vi "Get Reference.vi"(8 "Error In":errorcluster, 9 "Subpanel Ref":refnum<vi>, 11 "Sample Test Template in":refnum<class "Sample Test Template.lvclass">) -> (0 "Error Out":errorcluster, 3 "Sample Test Template out":refnum<class "Sample Test Template.lvclass">)   [LabVIEW 2020, in "Sample Test Template.lvclass"]
uses:
  Sample Test Template.lvclass
  D:/SDLC/Class/Test/Parent/Test.lvclass
  Parent/Typedef/LV2 Control.ctl
  Device/Parent/Device.lvclass
  Parent/Test.lvclass
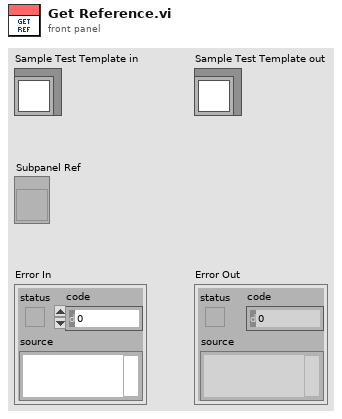
[diagram p1: front panel]
types:
  T1 = typedef "Test.lvclass/LV2 Control.ctl" = enum16{"Home", "Mode", "Config", "Status", "Read"}
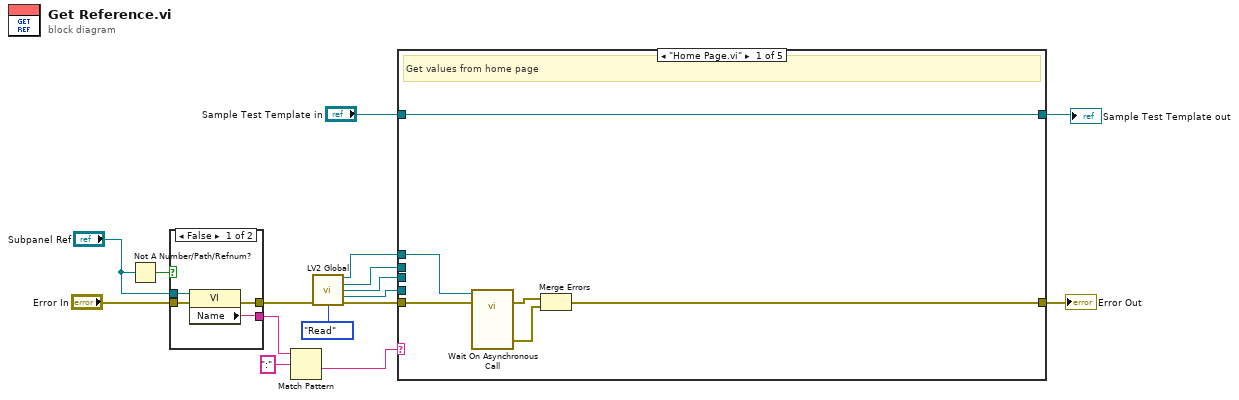
[diagram p0: block diagram]
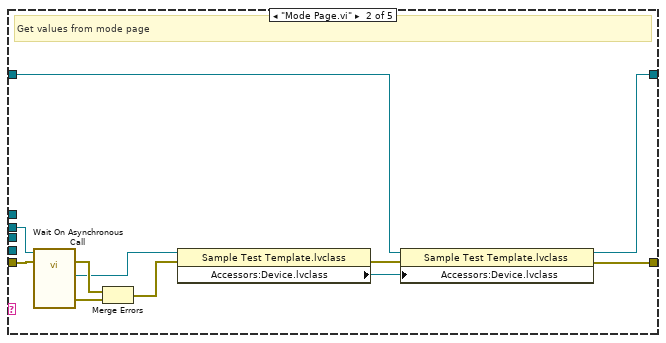
[diagram p2: hidden frame]
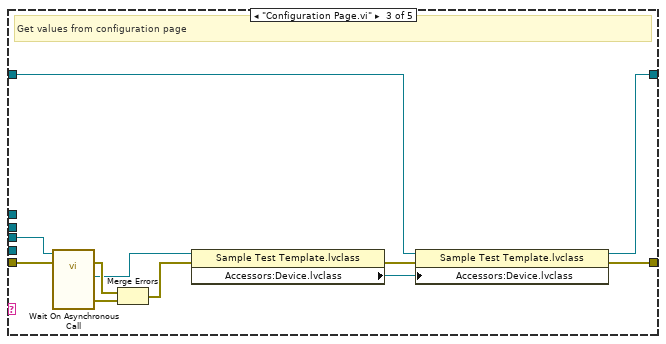
[diagram p3: hidden frame]
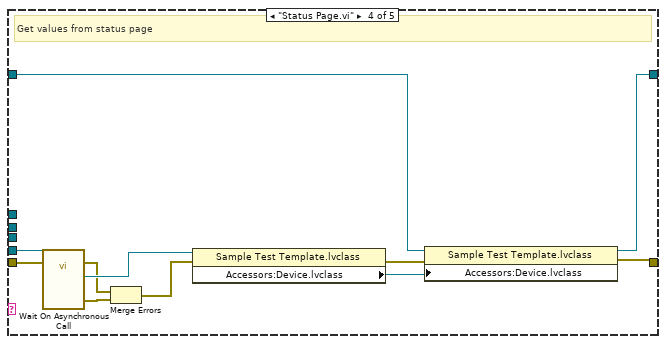
[diagram p4: hidden frame]
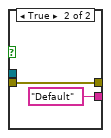
[diagram p6: hidden frame]
diagram:
  n1 = Not A Number/Path/Refnum?(number/path/refnum="Subpanel Ref") -> (NaN/Path/Refnum?=w16:bool)
  n2 = case shown="False" w16 {
    tunnel: "Error In" -> [w20 w22]
    tunnel: [w19 w22] -> w7
    tunnel: [w18 "Default" ("Name")] -> w15
    tunnel: "Subpanel Ref" -> [w17 _]
    frame False {
      n3 = property class="VI"(reference=w17, error in=w20) -> (error out=w19:errorcluster, "Name"=w18:string)  [unwired: 1 out]
    }
    frame True {
    }
  }
  n4 = Match Pattern(string=w15, regular expression=":") -> (after substring=w13:string)  [unwired: 1 in, 3 out]
  n5 = call "LV2 Global.vi"("Error In"=w7, "Enum"=LV2_Control."Read") -> ("Home Ref"=w1:refnum<vi>, "Mode Ref"=w4:refnum<vi>, "Configuration Ref"=w3:refnum<vi>, "Status Ref"=w2:refnum<vi>, "Error Out"=w6:errorcluster)  [unwired: 9 in]
  n6 = case shown="\"Home Page.vi\"" w13 {
    tunnel: w6 -> [w26 w39 w47 w61 w63]
    tunnel: [w23 w35 w43 w54 w63] -> w10
    tunnel: [w28 w30 w41 w52 w62] -> w8
    tunnel: "Sample Test Template in" -> [w28 w31 w42 w53 w62]
    tunnel: w4 -> [_ w29 _ _ _]
    tunnel: w3 -> [_ _ w40 _ _]
    tunnel: w2 -> [_ _ _ w51 _]
    tunnel: w1 -> [w27 _ _ _ _]
    frame "Home Page.vi" {
      # "Get values from home page"
      n7 = call-by-ref "Wait On Asynchronous Call"(reference=w27, error in=w26) -> (error out=w25:errorcluster, "Error Out"=w24:errorcluster)  [unwired: 14 in, 2 out]
      n8 = Merge Errors(w25, w24) -> (w23:errorcluster)
    }
    frame "Mode Page.vi" {
      # "Get values from mode page"
      n9 = call-by-ref "Wait On Asynchronous Call"(reference=w29, error in=w39) -> (error out=w38:errorcluster, 0:"error out"=w37:errorcluster, "Sample Test Template out"=w33:refnum<class "Sample Test Template.lvclass">)  [unwired: 10 in, 1 out]
      n10 = Merge Errors(w38, w37) -> (w36:errorcluster)
      n11 = property class="Sample Test Template.lvclass"(reference=w33, error in=w36) -> (error out=w34:errorcluster, "Accessors:Device.lvclass"=w32:refnum<class "Device.lvclass">)  [unwired: 1 out]
      n12 = property class="Sample Test Template.lvclass"(reference=w31, error in=w34, "Accessors:Device.lvclass"=w32) -> (reference out=w30:refnum<class "Sample Test Template.lvclass">, error out=w35:errorcluster)
    }
    frame "Configuration Page.vi" {
      # "Get values from configuration page"
      n13 = call-by-ref "Wait On Asynchronous Call"(reference=w40, error in=w47) -> (error out=w46:errorcluster, "Error Out"=w45:errorcluster, "Sample Test Template out"=w44:refnum<class "Sample Test Template.lvclass">)  [unwired: 10 in, 1 out]
      n14 = Merge Errors(w46, w45) -> (w50:errorcluster)
      n15 = property class="Sample Test Template.lvclass"(reference=w44, error in=w50) -> (error out=w49:errorcluster, "Accessors:Device.lvclass"=w48:refnum<class "Device.lvclass">)  [unwired: 1 out]
      n16 = property class="Sample Test Template.lvclass"(reference=w42, error in=w49, "Accessors:Device.lvclass"=w48) -> (reference out=w41:refnum<class "Sample Test Template.lvclass">, error out=w43:errorcluster)
    }
    frame "Status Page.vi" {
      # "Get values from status page"
      n17 = call-by-ref "Wait On Asynchronous Call"(reference=w51, error in=w61) -> (error out=w58:errorcluster, "Error Out"=w59:errorcluster, "Sample Test Template out"=w60:refnum<class "Sample Test Template.lvclass">)  [unwired: 10 in, 1 out]
      n18 = Merge Errors(w58, w59) -> (w57:errorcluster)
      n19 = property class="Sample Test Template.lvclass"(reference=w60, error in=w57) -> (error out=w56:errorcluster, "Accessors:Device.lvclass"=w55:refnum<class "Device.lvclass">)  [unwired: 1 out]
      n20 = property class="Sample Test Template.lvclass"(reference=w53, error in=w56, "Accessors:Device.lvclass"=w55) -> (reference out=w52:refnum<class "Sample Test Template.lvclass">, error out=w54:errorcluster)
    }
    frame Default {
      # "Default state"
    }
  }
  "Error Out" <- w10
  "Sample Test Template out" <- w8
